vi "libssh2_channel_open_ex.vi"(5 "packet_size":u32=32768, 7 "window_size":u32=2097152, 8 "error in (no error)":errorcluster, 9 "message":string, 10 "channel_type":string="session", 11 "Session":T1) -> (0 "error out":errorcluster, 3 "return value":u64)   [LabVIEW 2013, in "libssh2.lvlib"]
uses:
  libssh2.lvlib
  Session Refnum.ctl
  libssh2.dll
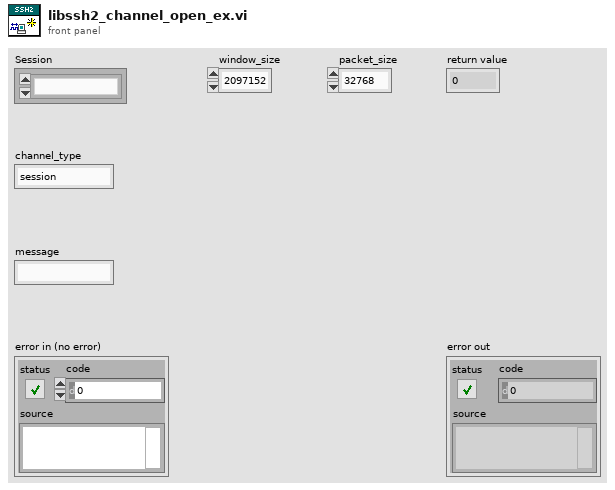
[diagram p1: front panel]
types:
  T1 = typedef "libssh2.lvlib/Session Refnum.ctl" = refnum<k1>
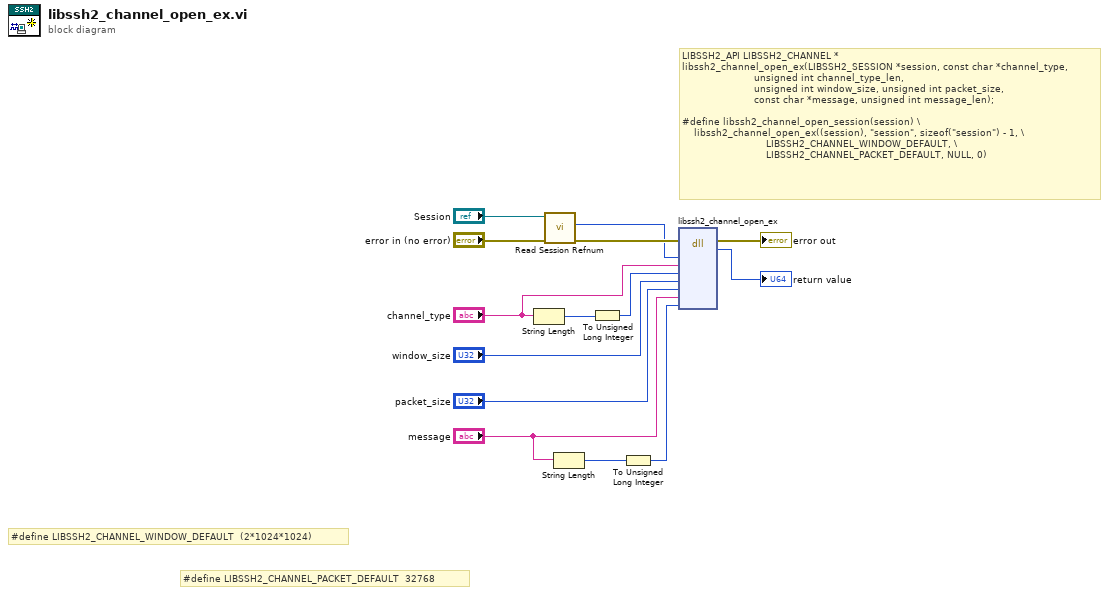
[diagram p0: block diagram]
diagram:
  # "#define LIBSSH2_CHANNEL_PACKET_DEFAULT  32768"
  # "#define LIBSSH2_CHANNEL_WINDOW_DEFAULT  (2*1024*1024)"
  # "LIBSSH2_API LIBSSH2_CHANNEL *\nlibssh2_channel_open_ex(LIBSSH2_SESSION *session, const char *channel_type,\n                        unsigned int channel_type_len,\n                        unsigned int window_size, unsigned int packet_size,\n                        const char *message, unsigned int message_len);\n\n#define libssh2_channel_open_session(session) \\\n    libssh2_channel_open_ex((session), \"session\", sizeof(\"session\") - 1, \\\n                            LIBSSH2_CHANNEL_WINDOW_DEFAULT, \\\n                            LIBSSH2_CHANNEL_PACKET_DEFAULT, NULL, 0)"
  n1 = String Length(string="channel_type") -> (length=w4:i32)
  n2 = call "Read Session Refnum.vi"("error in (no error)"="error in (no error)", "Session"="Session") -> ("error out"=w3:errorcluster, "LIBSSH2_SESSION*"=w1:u64)  [unwired: 8 in]
  n3 = String Length(string="message") -> (length=w5:i32)
  n4 = To Unsigned Long Integer(number=w4) -> (unsigned 32bit integer=w14:u32)
  n5 = To Unsigned Long Integer(number=w5) -> (unsigned 32bit integer=w7:u32)
  n6 = dll-call lib="C:/Users/pasca/source/repos/libssh2-labview/libssh2**.*" fn="libssh2_channel_open_ex"(error in=w3, "session"=w1, "channel_type"="channel_type", "channel_type_len"=w14, "window_size"="window_size", "packet_size"="packet_size", "message"="message", "message_len"=w7) -> (error out=→"error out":errorcluster, "return value"=→"return value":u64)  [unwired: 9 in, 1 out]
